vi "prepAI_focusalign.vi"(3 "rate":dbl=30000.0 format="%#_13g", 4 "bufferAI":i32, 5 "triggersource":tag) -> (0 "error out":errorcluster, 1 "header":dbl[](array[numeric]), 2 "task out":refnum<k21>)   [LabVIEW 2015]
uses:
  <vilib>/DAQmx/create/channels.llb/DAQmx Create Channel (AI-Voltage-Basic).vi
  <vilib>/DAQmx/configure/timing.llb/DAQmx Timing (Sample Clock).vi
  <vilib>/DAQmx/configure/trigger.llb/DAQmx Start Trigger (Digital Edge).vi
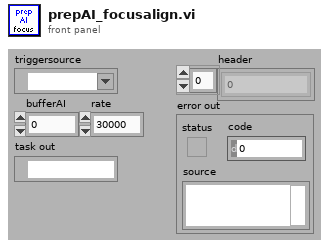
[diagram p1: front panel]
types:
  T1 = cluster{"StageS":i32, "StageL":i32, "currmeas data dir":path, "image OD":u16, "contour OD":u16, "point OD":u16, "AOlines":tag[], "AIlines":tag[], "CI lines":tag[], "DO lines":tag[], "AO names":string[], "CI names":string[], "AI names":string[], "DO names":string[], "CIextensions":string[], "AIextensions":string[], "Voltage to Ygalvo":i32, "Voltage to Xgalvo":i32, "Voltage to patch":i32, "640 shutter":i32, "2P shutter":i32, "LT timestamp":u32, "Vp":i32, "Ip":i32, "camera trigger":i32, "master data dir":path, "voltage to Zpos":i32, "Vto2P":i32, "640 AO":i32, "488 AO":i32, "532 AO":i32, "640TTL":u32, "488TTL":u32, "532TTL":u32, "Device 1 sampleclock out":tag, "Device 1 Starttrigger out":tag, "Device 2 sampleclock in":tag, "Device 2 StartTrigger in ":tag, "2PODTTL":u32, "488 shutter":u32, "LCVR red":u32, "LCVR blue":u32}
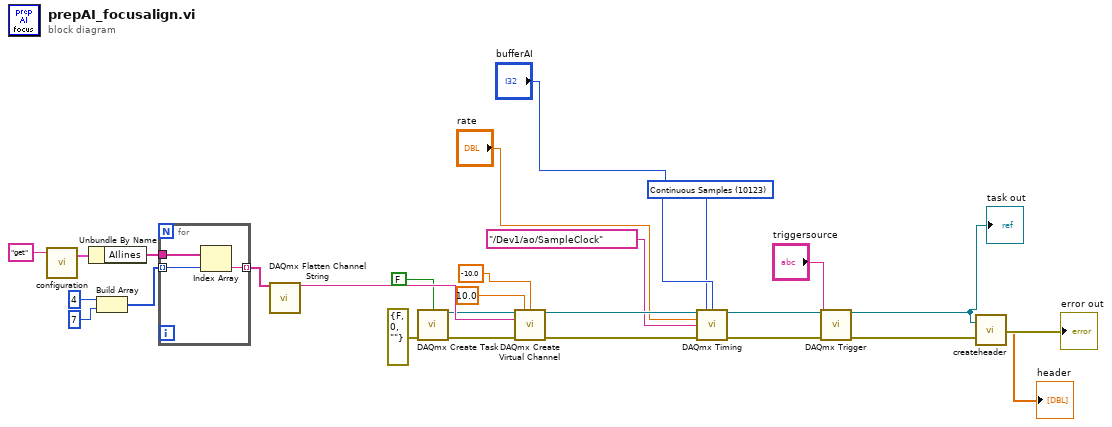
[diagram p0: block diagram]
diagram:
  w5 = 10123 items=["Finite Samples"=10178, "Continuous Samples"=10123, "Hardware Timed Single Point"=12522] ("sample mode")
  n1 = call "configuration.vi"("command"="get") -> ("config out"=w26:T1)  [unwired: 2 in, 1 out]
  n2 = Unbundle By Name(w26) -> ("AIlines"=w25:tag[])
  n3 = Build Array(4, 7) -> (w20:i32[])
  n4 = for {
    tunnel: w20 -> [w30] mode=indexing
    tunnel: w25 -> [w29]
    tunnel: [w28] -> w1 mode=indexing
    n5 = Index Array(array=w29, index=w30) -> (element=w28:tag)
  }
  n6 = call <vilib>:"DAQmx Flatten Channel String.vi"("names in"=w1) -> ("names out"=w24:string)  [unwired: 13 in, 1 out]
  n7 = call <vilib>:"DAQmx Create Task.vi"("auto cleanup"=FALSE, "error in"=errorcluster {"status"=FALSE, "code"=0, "source"=""}) -> ("task out"=w9:refnum<k21>, "error out"=w10:errorcluster)  [unwired: 12 in]
  n8 = call-poly <vilib>:"DAQmx Create Virtual Channel.vi"("task in"=w9, "maximum value"=10.0, "minimum value"=-10.0, "physical channels"=w24, "error in"=w10) -> ("task out"=w19:refnum<k21>, "error out"=w18:errorcluster)  [unwired: 9 in]
  n9 = call-poly <vilib>:"DAQmx Timing.vi"("task/channels in"=w19, "sample mode"=w5, "samples per channel"="bufferAI", "rate"="rate", "source"=tag "/Dev1/ao/SampleClock", "error in"=w18) -> ("task out"=w14:refnum<k21>, "error out"=w8:errorcluster)  [unwired: 8 in]
  n10 = call-poly <vilib>:"DAQmx Trigger.vi"("task/channels in"=w14, "source"="triggersource", "error in"=w8) -> ("task out"=w3:refnum<k21>, "error out"=w7:errorcluster)  [unwired: 11 in]
  "task out" <- w3
  n11 = call "createheader.vi"("task in"=w3, "error in"=w7) -> ("Array"=→"header":dbl[], "error out"=→"error out":errorcluster)  [unwired: 1 out]
